vi "Close_Device.vi"(2 "error in":errorcluster, 3 "Device Session":refnum<visa-resource-name>) -> (0 "error out":errorcluster)   [LabVIEW 2017]
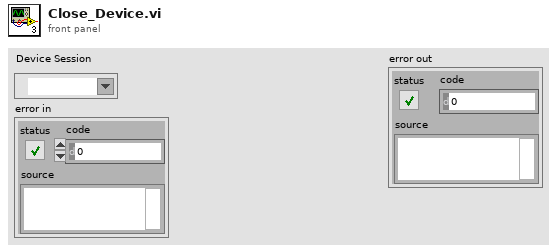
[diagram p1: front panel]
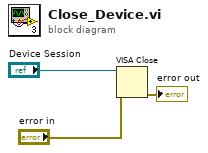
[diagram p0: block diagram]
diagram:
  n1 = VISA Close(VISA resource name="Device Session", error in (no error)="error in") -> (error out=→"error out":errorcluster)
